vi "Format CMD for Log.vi"(3 "error in":errorcluster, 5 "Command":T1) -> (0 "error out":errorcluster, 1 "Stim CMD for Log":string, 2 "Command":T1)   [LabVIEW 2019]
uses:
  Bits Library/Get Bits (U8).vi
  Bits Library/Get Bit (U8).vi
  Bits Library/Bits.lvlib
panel:
  out "Command Name":string
  out "String":string
  out "1st byte":u8 format="%b"
  out "Cmd string byte array":u8[](array[numeric]) format="%08b"
  # "These should match"
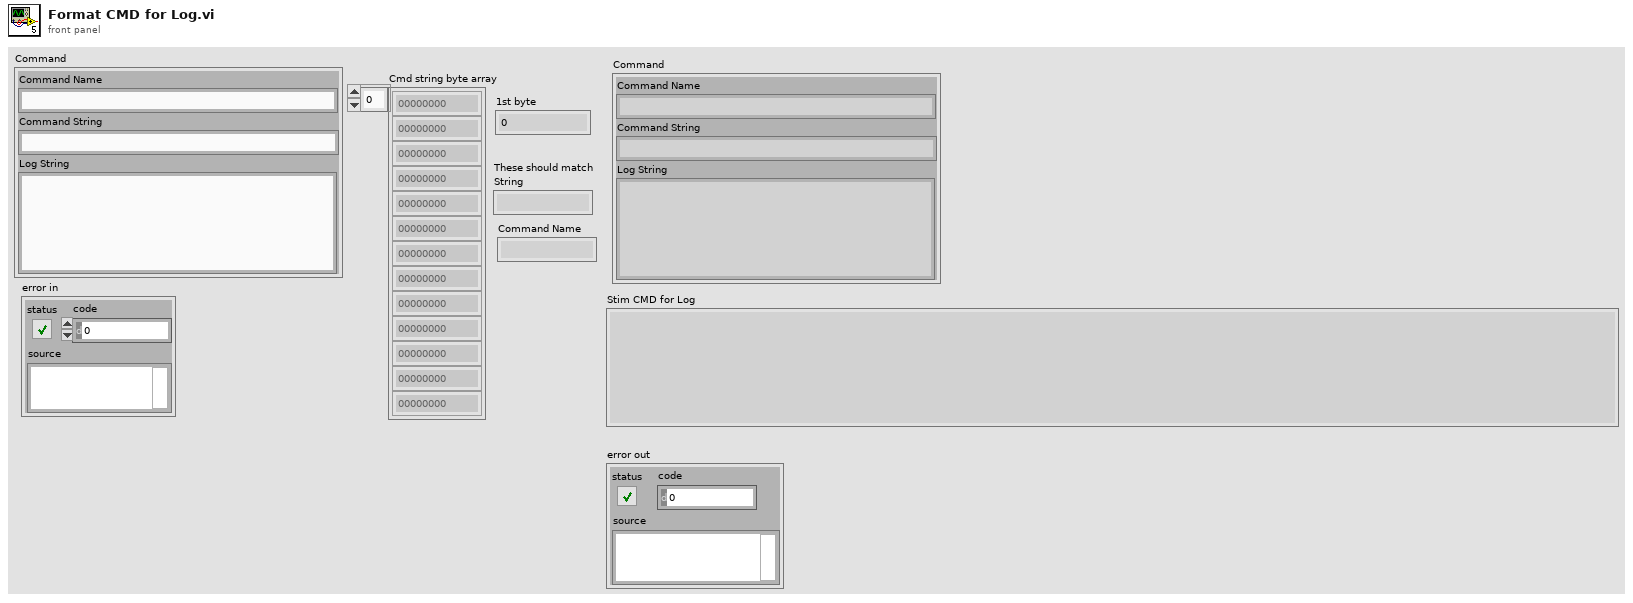
[diagram p1: front panel]
types:
  T1 = cluster{"Command Name":string, "Command String":string, "Log String":string}
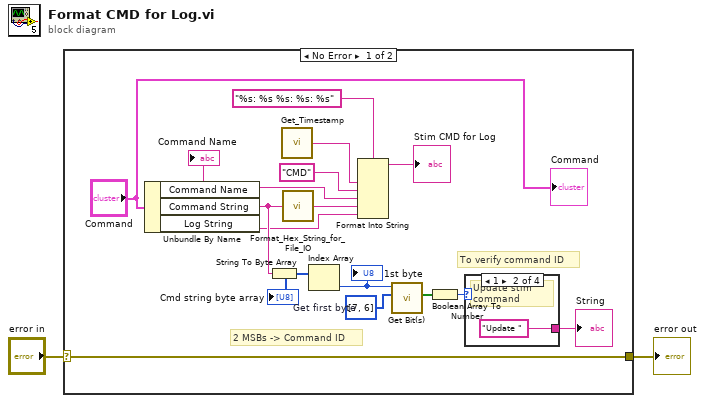
[diagram p0: block diagram]
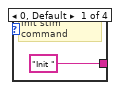
[diagram p2: hidden frame]
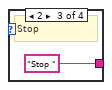
[diagram p3: hidden frame]
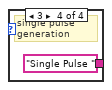
[diagram p4: hidden frame]
diagram:
  n1 = case shown="No Error" "error in" {
    selector: "error in" -> [w17 w23]
    tunnel: [w17 w23] -> w1
    frame No Error {
      # "To verify command ID"
      # "2 MSBs -> Command ID"
      n2 = Unbundle By Name("Command") -> ("Command Name"=w10:string, "Command String"=w8:string, "Log String"=w3:string)
      "Command Name" <- w10
      n3 = String To Byte Array(string=w8) -> (unsigned byte array=w16:u8[])
      "Cmd string byte array" <- w16
      n4 = call "Get_Timestamp.vi"() -> ("date/time string"=w5:string)  [unwired: 1 in]
      n5 = call "Format_Hex_String_for_File_IO.vi"("Hex String in"=w8) -> ("Hex String out"=w7:string)
      n6 = Index Array "Get first byte"(array=w16) -> (element=w12:u8)  [unwired: 1 in]
      "1st byte" <- w12
      n7 = Format Into String(format string="%s: %s %s: %s: %s", w5, "CMD" ("input 1"), w10, w7, w3) -> (resulting string=→"Stim CMD for Log":string)  [unwired: 2 in, 1 out]
      n8 = call-poly "Get Bit(s).vi"("Bits"=u8[] [7, 6], "Number"=w12) -> ("Values"=w14:bool[])  [unwired: 8 in, 1 out]
      n9 = Boolean Array To Number(Boolean array=w14) -> (number=w13:u32)
      n10 = case shown="1" w13 {
        tunnel: ["Init " "Update " "Stop " "Single Pulse "] -> w11
        frame 0, Default {
          # "Init stim command"
        }
        frame 1 {
          # "Update stim command"
        }
        frame 2 {
          # "Stop"
        }
        frame 3 {
          # "single pulse generation"
        }
      }
      "String" <- w11
      "Command" <- "Command"
    }
    frame Error {
    }
  }
  "error out" <- w1
